vi "clone.vi"(0 "reference":refnum<class "AbstractEdge.lvclass">, 5 "error in (no error)":errorcluster) -> (14 "reference out":refnum<class "AbstractEdge.lvclass">, 15 "clonedEdge":refnum<class "AbstractEdge.lvclass">, 19 "error out":errorcluster)   [LabVIEW 2020, in "AbstractEdge.lvclass"]
doc: "public Object clone()"
uses:
  <resource>/Framework/Providers/Open_GDS/UML/AbstractEdge_class/AbstractEdge.lvclass
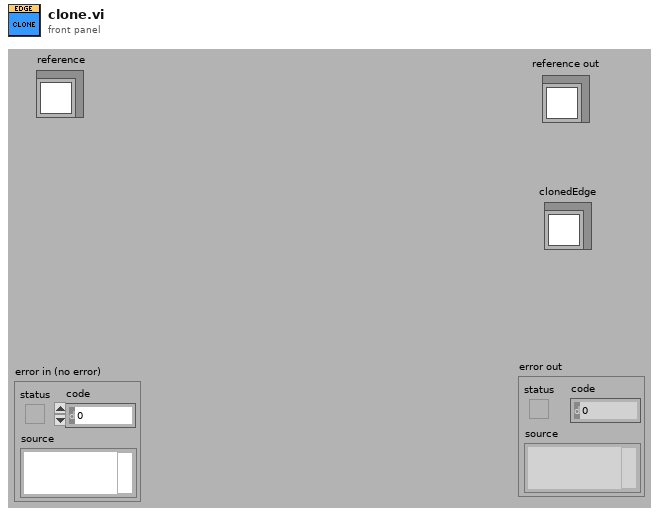
[diagram p1: front panel]
types:
  T1 = typedef "AbstractEdge.lvclass/ObjectAttributes.ctl" = cluster{"start":refnum<class "AbstractNode.lvclass">, "end":refnum<class "AbstractNode.lvclass">}
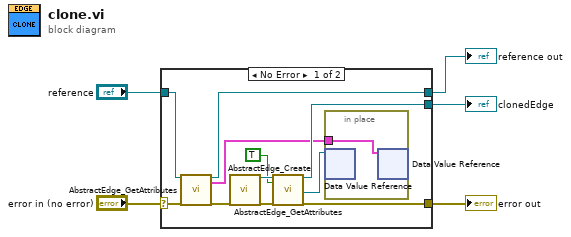
[diagram p0: block diagram]
diagram:
  n1 = case shown="No Error" "error in (no error)" {
    selector: "error in (no error)" -> [w13 w18]
    tunnel: "reference" -> [w16 w19]
    tunnel: [w15 w18] -> w4
    tunnel: [w14 w19] -> w3
    tunnel: [w12 _] -> w1
    frame No Error {
      n2 = call <resource>:"AbstractEdge_GetAttributes.vi"("reference in"=w16, "error in (no error)"=w13) -> ("reference out"=w14:refnum<class "AbstractEdge.lvclass">, "Data"=w6:T1, "error out"=w9:errorcluster)  [unwired: 1 in, 14 out]
      n3 = call <resource>:"AbstractEdge_Create.vi"("error in (no error)"=w9) -> ("reference out"=w11:refnum<class "AbstractEdge.lvclass">, "error out"=w10:errorcluster)  [unwired: 1 in, 16 out]
      n4 = call <resource>:"AbstractEdge_GetAttributes.vi"("reference in"=w11, "OnlyGetDvrReference(False)"=TRUE, "error in (no error)"=w10) -> ("reference out"=w12:refnum<class "AbstractEdge.lvclass">, "DataRef"=w7:refnum<data-value>, "error out"=w15:errorcluster)  [unwired: 13 in, 1 out]
      n5 = in-place {
        in-place-border: w6 -> [w17]
        n6 = in-place-dvr #1(w7) -> ()  [unwired: 2 out]
        n7 = in-place-dvr #1(w17) -> ()  [unwired: 2 out]
      }
    }
    frame Error {
    }
  }
  "reference out" <- w3
  "error out" <- w4
  "clonedEdge" <- w1
